vi "Inter-Move Items (inline).vi"(4 "indent":i32, 6 "Insertion index":i32, 7 "BetterHandle in (source)":refnum<class "BetterHandle.lvclass">, 8 "error in (no error)":errorcluster, 9 "Copy?":bool, 10 "Indices to move":i32[](array[numeric]), 11 "BetterHandle in (destination)":refnum<class "BetterHandle.lvclass">) -> (0 "error out":errorcluster, 3 "BetterHandle out (destination)":refnum<class "BetterHandle.lvclass">, 5 "BetterHandle out (source)":refnum<class "BetterHandle.lvclass">)   [LabVIEW 2020, in "BetterDragAndDrop.lvlib" / "BetterHandle.lvclass"]
uses:
  BetterHandle.lvclass
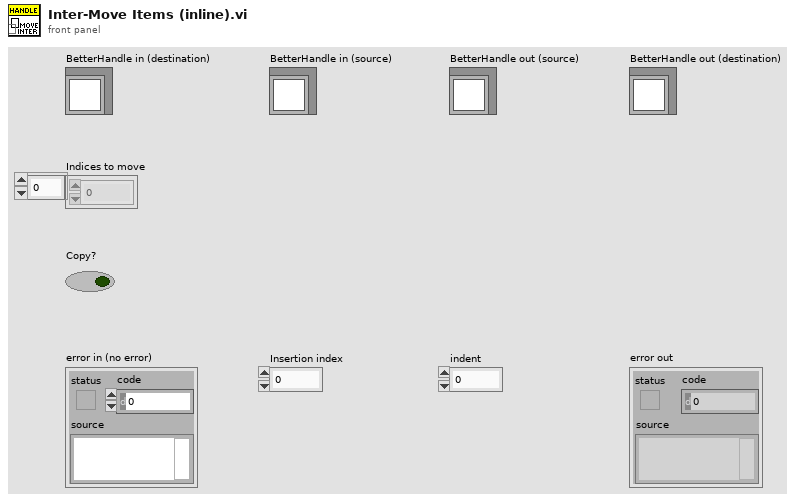
[diagram p1: front panel]
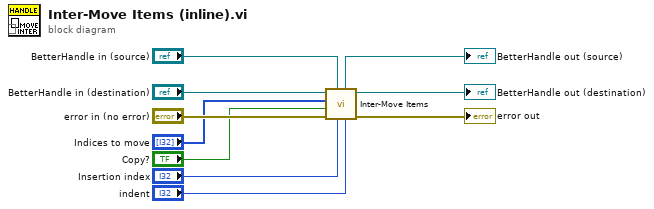
[diagram p0: block diagram]
diagram:
  n1 = call "Inter-Move Items.vi"("indent"="indent", "Insertion index"="Insertion index", "BetterHandle in (source)"="BetterHandle in (source)", "error in (no error)"="error in (no error)", "Copy?"="Copy?", "Indices to move"="Indices to move", "BetterHandle in (destination)"="BetterHandle in (destination)") -> ("error out"=→"error out":errorcluster, "BetterHandle out (destination)"=→"BetterHandle out (destination)":refnum<class "BetterHandle.lvclass">, "BetterHandle out (source)"=→"BetterHandle out (source)":refnum<class "BetterHandle.lvclass">)  [unwired: 2 in]
